vi "PatMat_first2frames.vi"() -> ()   [LabVIEW 2012]
uses:
  <vilib>/imath/engines/lvmath2/RunTimeEngine/NodeEndStatement/NIMS_NodeEndStatement_Output.vi
  <instcachedir>/0/NIMS_NodeEndStatement_Output_53EC0D466D134D7ABD903AC30B43404B.lvgen/NIMS_NodeEndStatement_Output_53EC0D466D134D7ABD903AC30B43404B_001.vi
  <instcachedir>/0/NIMS_NodeEndStatement_Output_53EC0D466D134D7ABD903AC30B43404B.lvgen/NIMS_NodeEndStatement_Output_53EC0D466D134D7ABD903AC30B43404B_005.vi
  <vilib>/imath/engines/lvmath2/RunTimeEngine/ErrorHandling/NIMS_Finalize Error.vi
  <vilib>/Utility/file.llb/Write To Spreadsheet File (I64).vi
panel:
  out "Delta_Y (TempBox-Template)":dbl
  out "Delta_X (TempBox-Template)":dbl
  out "Matched TempBox (y,x)":i32[](array[numeric])
  out "Min_SAD":u32
  out "SAD":u32[][](array[numeric])
  in  "Template \n      in \n1st frame\n    s_y":dbl=282.0
  in  "Template \n      in \n1st frame\n    e_y":dbl=291.0
  in  "Template \n      in \n1st frame\n    e_x":dbl=692.0
  in  "Template \n      in\n1st frame\n     s_x":dbl=658.0
  in  "ROI in\n2nd frame\n    e_y":dbl=301.0
  in  "ROI in\n2nd frame\n    s_y":dbl=272.0
  in  "ROI in\n2nd frame\n    e_x":dbl=727.0
  in  "ROI in\n2nd frame\n    s_x":dbl=623.0
  in  "1st frame":dbl=153.0
  in  "?":bool
  out "Template in 1st frame":u8[][](array[numeric])
  out "Frames":T1(plugin-control)
  out "framesPerSecond":u32
  out "Image Type":T2 items=["Grayscale (U8)", "Grayscale (I16)", "Grayscale (SGL)", "Complex (CSG)", "RGB (U32)", "HSL (U32)", "RGB (U64)"]
  out "Number of Frames":u32
  in  "Path":path=path "C:/Users/admin/Desktop/lohit/pat3.avi"
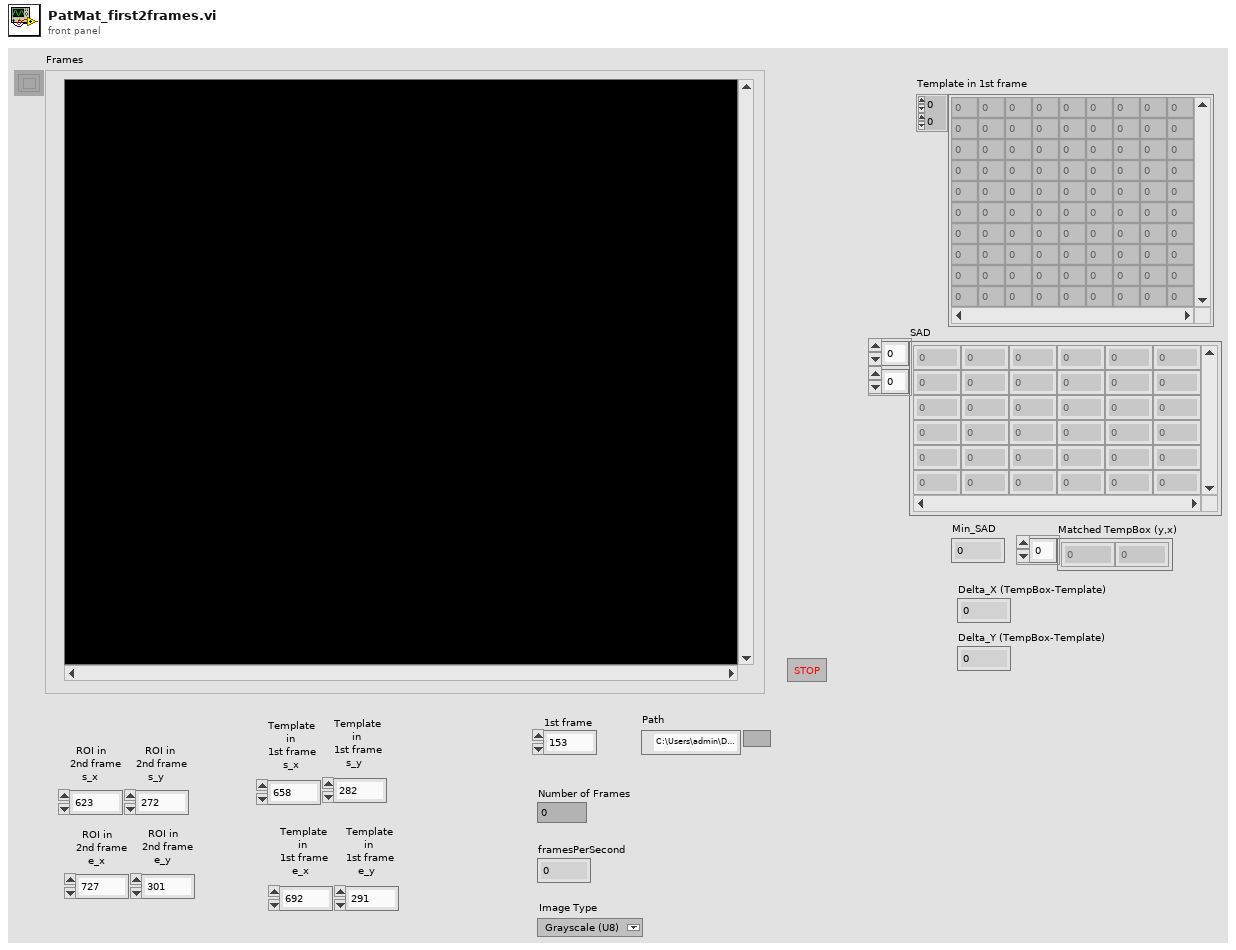
[diagram p1: front panel]
types:
  T1 = typedef "IMAQ Image.ctl" = refnum<image>
  T2 = typedef "Image Type" = u32
  T3 = typedef "AviRefnum.ctl" = refnum<k1>
  T4 = cluster{"width":u32, "height":u32, "framesPerSecond":u32, "compressionFilter":string, "hasData":bool}
  T5 = cluster{"[0]":i32, "[1]":i32, "[2]":i32, "[3]":i32, "[4]":i32, "[5]":i32, "[6]":i32, "[7]":i32, "[8]":i32}
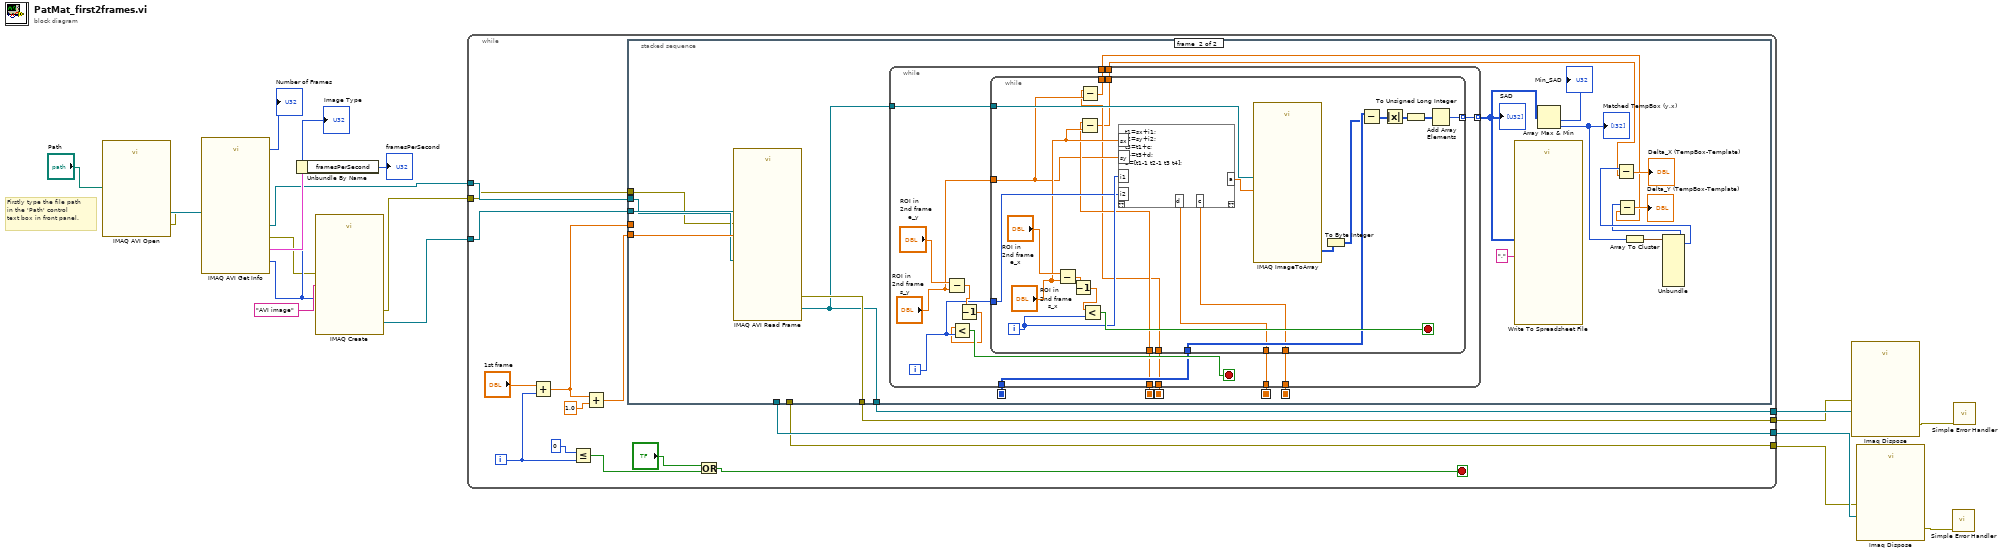
[diagram p0: block diagram]
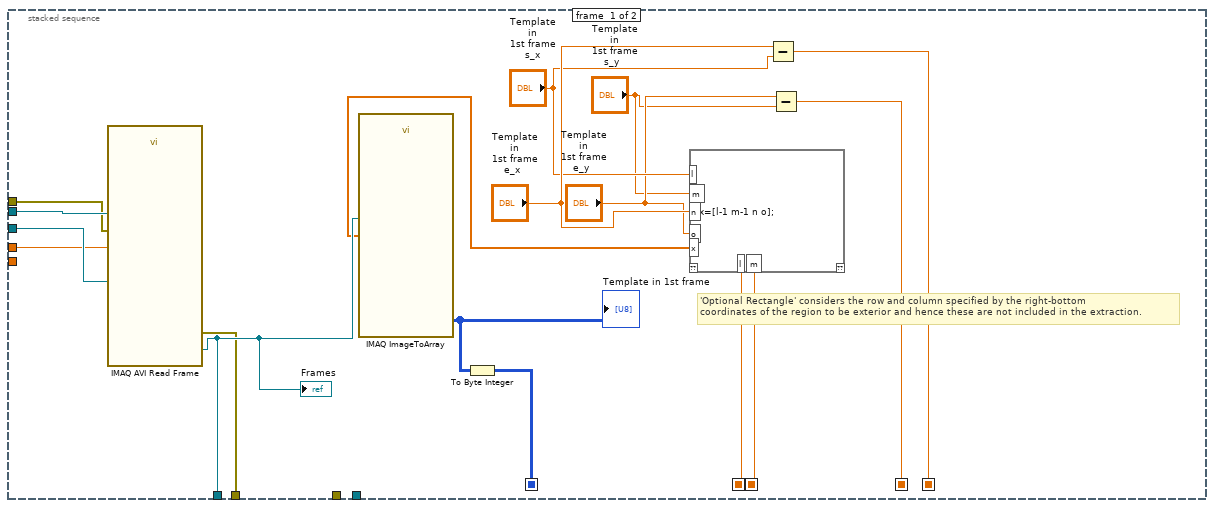
[diagram p2: hidden frame]
diagram:
  # "Firstly type the file path\nin the 'Path' control \ntext box in front panel."
  n1 = call "IMAQ AVI Open"("AVI Path"="Path") -> ("error out"=w11:errorcluster, "Avi Refnum"=w17:T3)  [unwired: 9 in]
  n2 = call "IMAQ AVI Get Info"("error in (no error)"=w11, "Avi Refnum"=w17) -> ("error out"=w10:errorcluster, "Image Type"=w13:T2, "Number of Frames"=→"Number of Frames":u32, "Avi Refnum (duplicate)"=w9:T3, "Frame Data"=w15:T4)  [unwired: 5 in]
  "Image Type" <- w13
  n3 = Unbundle By Name(w15) -> ("framesPerSecond"=→"framesPerSecond":u32)
  n4 = call "IMAQ Create"("Image Name"="AVI image", "Image Type"=w13, "error in (no error)"=w10) -> ("New Image"=w7:T1, "error out"=w8:errorcluster)  [unwired: 2 in]
  n5 = while {
    tunnel: w9 -> [w30]
    tunnel: w8 -> [w29]
    tunnel: w7 -> [w28]
    tunnel: [w23] -> w5
    tunnel: [w22] -> w4
    tunnel: [w21] -> w3
    tunnel: [w20] -> w2
    i -> [w32]
    stop <- w33 stop-if-true
    n6 = Add(x="1st frame", y=w32) -> (x+y=w27:dbl)
    n7 = Less Or Equal?(x=0, y=w32) -> (x <= y?=w25:bool)
    n8 = Add(x=w27, y=1.0) -> (x+y=w26:dbl)
    n9 = stacked-sequence {
      seq-local: [w46 _] -> [_ w100]
      seq-local: [w37 _] -> [_ w98]
      seq-local: [w38 _] -> [_ w99]
      seq-local: [w36 _] -> [_ w94]
      seq-local: [w35 _] -> [_ w93]
      tunnel: w30 -> [w50 w105]
      tunnel: w29 -> [w49 w103]
      tunnel: w28 -> [w48 w104]
      tunnel: w27 -> [w47 _]
      tunnel: w26 -> [_ w106]
      tunnel: [_ w101] -> w23
      tunnel: [w45 _] -> w22
      tunnel: [w44 _] -> w21
      tunnel: [_ w102] -> w20
      frame #0 {
        # "'Optional Rectangle' considers the row and column specified by the right-bottom\ncoordinates of the region to be exterior and hence these are not included in the extraction."
        n10 = call "IMAQ AVI Read Frame"("error in (no error)"=w49, "Frame Number"=w47, "Image"=w48, "Avi Refnum"=w50) -> ("error out"=w44:errorcluster, "Image Out"=w45:T1)  [unwired: 4 in, 2 out]
        "Frames" <- w45
        n11 = mathscript code="x=[l-1 m-1 n o];"("l"="Template \n      in\n1st frame\n     s_x", "m"="Template \n      in \n1st frame\n    s_y", "n"="Template \n      in \n1st frame\n    e_x", "o"="Template \n      in \n1st frame\n    e_y") -> ("x"=w43:dbl[], "l"=w36:dbl, "m"=w35:dbl)  [unwired: 1 in, 1 out]
        n12 = call "IMAQ ImageToArray"("Optional Rectangle"=w43, "Image"=w45) -> ("Image Pixels (U8)"=w51:u8[][])  [unwired: 2 in, 4 out]
        "Template in 1st frame" <- w51
        n13 = To Byte Integer(number=w51) -> (8bit integer=w46:i8[][])
        n14 = Subtract(x="Template \n      in \n1st frame\n    e_x", y="Template \n      in\n1st frame\n     s_x") -> (x-y=w38:dbl)
        n15 = Subtract(x="Template \n      in \n1st frame\n    e_y", y="Template \n      in \n1st frame\n    s_y") -> (x-y=w37:dbl)
      }
      frame #1 {
        n16 = call "IMAQ AVI Read Frame"("error in (no error)"=w103, "Frame Number"=w106, "Image"=w104, "Avi Refnum"=w105) -> ("error out"=w102:errorcluster, "Image Out"=w101:T1)  [unwired: 4 in, 2 out]
        n17 = while {
          tunnel: w101 -> [w119]
          tunnel: w100 -> [w117]
          tunnel: w99 -> [w114]
          tunnel: w98 -> [w113]
          tunnel: [w112] -> w96 mode=indexing
          tunnel: w94 -> [w111]
          tunnel: w93 -> [w110]
          tunnel: [w109] -> w87
          tunnel: [w108] -> w85
          i -> [w118]
          stop <- w120 stop-if-true
          n18 = Subtract(x="ROI in\n2nd frame\n    e_y", y="ROI in\n2nd frame\n    s_y") -> (x-y=w121:dbl)
          n19 = Decrement(x=w121) -> (x-1=w107:dbl)
          n20 = Less?(x=w107, y=w118) -> (x < y?=w120:bool)
          n21 = while {
            tunnel: w119 -> [w141]
            tunnel: "ROI in\n2nd frame\n    s_y" -> [w126]
            tunnel: w118 -> [w139]
            tunnel: w117 -> [w134]
            tunnel: w114 -> [w131]
            tunnel: w113 -> [w130]
            tunnel: [w129] -> w112 mode=indexing
            tunnel: w111 -> [w127]
            tunnel: w110 -> [w125]
            tunnel: [w124] -> w109
            tunnel: [w123] -> w108
            i -> [w140]
            stop <- w142 stop-if-true
            n22 = Subtract(x="ROI in\n2nd frame\n    e_x", y="ROI in\n2nd frame\n    s_x") -> (x-y=w143:dbl)
            n23 = Decrement(x=w143) -> (x-1=w122:dbl)
            n24 = Subtract(x=w127, y="ROI in\n2nd frame\n    s_x") -> (x-y=w124:dbl)
            n25 = Subtract(x=w125, y=w126) -> (x-y=w123:dbl)
            n26 = Less?(x=w122, y=w140) -> (x < y?=w142:bool)
            n27 = mathscript code="t1=sx+i1;\nt2=sy+i2;\nt3=t1+c;\nt4=t3+d;\na=[t1-1 t2-1 t3 t4];"("sx"="ROI in\n2nd frame\n    s_x", "sy"=w126, "i1"=w140, "i2"=w139, "c"=w131, "d"=w130) -> ("a"=w138:dbl[])  [unwired: 1 in, 1 out]
            n28 = call "IMAQ ImageToArray"("Optional Rectangle"=w138, "Image"=w141) -> ("Image Pixels (U8)"=w144:u8[][])  [unwired: 2 in, 4 out]
            n29 = To Byte Integer(number=w144) -> (8bit integer=w133:i8[][])
            n30 = Subtract(x=w134, y=w133) -> (x-y=w136:i8[][])
            n31 = Absolute Value(x=w136) -> (abs(x)=w135:i8[][])
            n32 = To Unsigned Long Integer(number=w135) -> (unsigned 32bit integer=w137:u32[][])
            n33 = Add Array Elements(numeric array=w137) -> (sum=w129:u32)
          }
        }
        "SAD" <- w96
        n34 = call-poly <vilib>:"Write To Spreadsheet File.vi"("delimiter (\\t)"="," ("delimiter (\\t)"), "2D data"=w96) -> ()  [unwired: 6 in, 1 out]
        n35 = Array Max & Min(array=w96) -> (min value=→"Min_SAD":u32, min index (indices)=w92:i32[])  [unwired: 2 out]
        "Matched TempBox (y,x)" <- w92
        n36 = Array To Cluster(array=w92) -> (cluster=w91:T5)
        n37 = Unbundle(w91) -> ("[0]"=w86:i32, "[1]"=w88:i32)  [unwired: 7 out]
        n38 = Subtract(x=w88, y=w87) -> (x-y=→"Delta_X (TempBox-Template)":dbl)
        n39 = Subtract(x=w86, y=w85) -> (x-y=→"Delta_Y (TempBox-Template)":dbl)
      }
    }
    n40 = Or(x="?", y=w25) -> (x .or. y?=w33:bool)
  }
  n41 = call "Imaq Dispose"("Image"=w5, "error in (no error)"=w2) -> ("error out"=w6:errorcluster)  [unwired: 4 in]
  n42 = call "Imaq Dispose"("Image"=w4, "error in (no error)"=w3) -> ("error out"=w1:errorcluster)  [unwired: 4 in]
  n43 = call <vilib>:"Simple Error Handler.vi"("error in (no error)"=w1) -> ()  [unwired: 4 in, 5 out]
  n44 = call <vilib>:"Simple Error Handler.vi"("error in (no error)"=w6) -> ()  [unwired: 4 in, 5 out]
